vi "CVT String GetIndex.vi"(8 "error in (no error)":errorcluster, 11 "Tag Name":string) -> (0 "error out":errorcluster, 3 "Tag Index":i32)   [LabVIEW 2010]
uses:
  _SubVIs/TypeDefs/cvt_TagList Methods.ctl
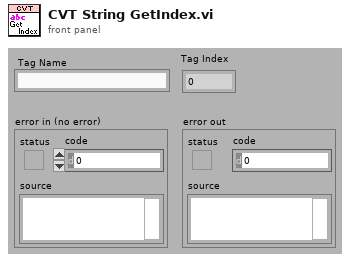
[diagram p1: front panel]
types:
  T1 = typedef "cvt_TagList Methods.ctl" = enum16{"init", "getindex", "getdesc", "getlist"}
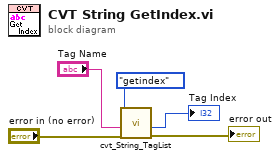
[diagram p0: block diagram]
diagram:
  n1 = call "cvt_String_TagList.vi"("error in (no error)"="error in (no error)", "Tag Name"="Tag Name", "Method"=cvt_TagList_Methods."getindex") -> ("error out"=→"error out":errorcluster, "Index"=→"Tag Index":i32)  [unwired: 1 in, 6 out]
